vi "例4.6.vi"() -> ()   [LabVIEW 2018]
panel:
  out "x":dbl
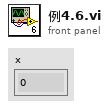
[diagram p1: front panel]
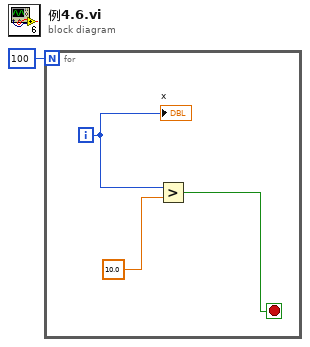
[diagram p0: block diagram]
diagram:
  n1 = for {
    N: 100 -> [_]
    i -> [w3]
    stop <- w2 stop-if-true
    n2 = Greater?(x=w3, y=10.0) -> (0:w2:bool)
    "x" <- w3
  }
